vi "_FPGA Check Turbo.vi"(4 "error in":errorcluster) -> (0 "error out":errorcluster, 2 "SpeedOK":bool)   [LabVIEW 2015]
uses:
  Type/_Pump Parameter.ctl
  _RT Global.vi
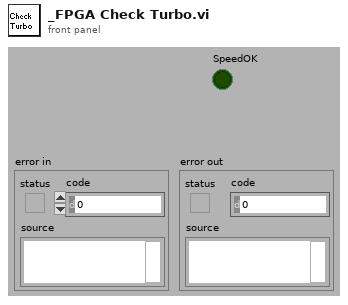
[diagram p1: front panel]
types:
  T1 = typedef "_Pump Parameter.ctl" = enum16{"Turn Pump Motor On", "Turn Pump Motor Off", "Read Pump Oil Deficiency", "Read Rotation Switch Point Attained", "Read Ele. Drive Over Temperature", "Read Pump Over Temperature", "Read Set Rotation Speed Attained", "Read Turbopump Accelerates", "Read Actual Rotation Speed in Hz", "Read Motor Current in A", "Read Operating Hours in h", "Read Motor Voltage in V", "Read Motor Power in W", "Set Rotation Speed Switchpoint in %", "Clear Error", "Read Error Code", "Read Bearing Temperature", "Read Hardware Version", "Read Firmware Version", "Read Operating Hours (Drive)", "Read Rotational Speed (rpm)", "Read Power Stage Temperature", "Read Electronics Temperature", "Read Upper Pump Temperature", "Read Motor Temperature", "Read Error Code History, 1", "Read Error Code History, 2", "Read Error Code History, 3", "Read Error Code History, 4", "Read Error Code History, 5", "Read Error Code History, 6", "Read Error Code History, 7", "Read Error Code History, 8", "Read Error Code History, 9", "Read Error Code History, 10"}
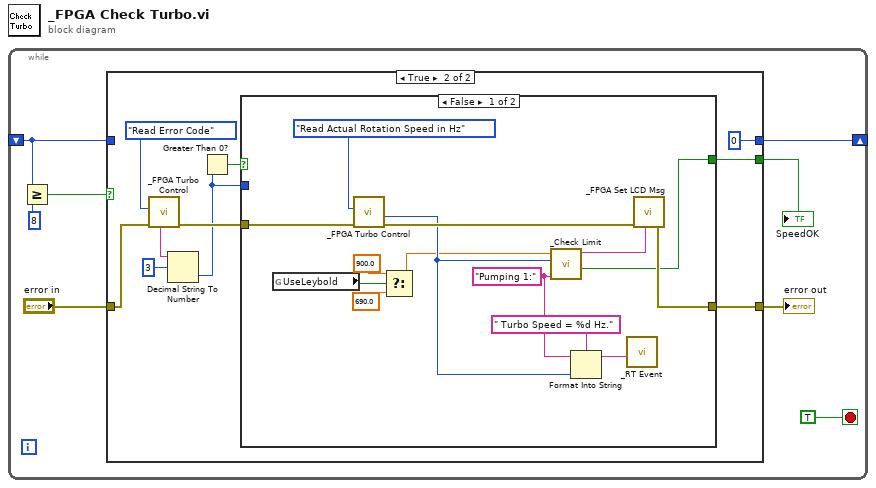
[diagram p0: block diagram]
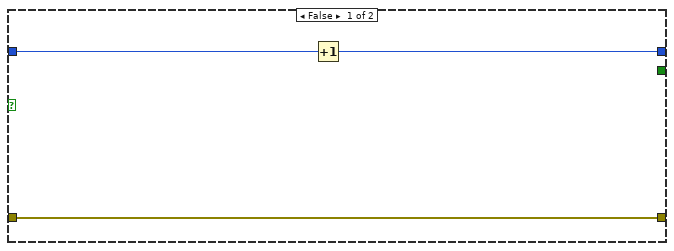
[diagram p2: hidden frame]
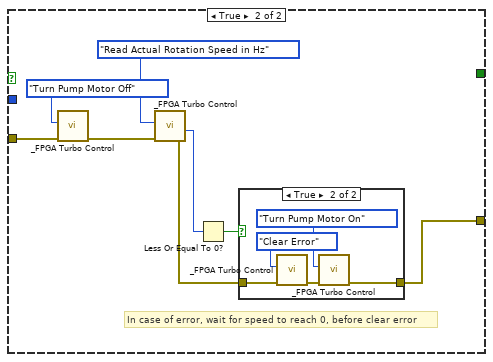
[diagram p3: hidden frame]
diagram:
  n1 = while {
    shift-right: [w7] -> _
    shift-left: _ -> [w5]
    stop <- TRUE stop-if-true
    n2 = Greater Or Equal?(x=w5, y=8) -> (x >= y?=w1:bool)
    n3 = case shown="True" w1 {
      tunnel: [w10 0] -> w7
      tunnel: w5 -> [w11 _]
      tunnel: [w9 w20] -> w3
      tunnel: "error in" -> [w9 w18]
      tunnel: [_ w19] -> w2
      frame False {
        n4 = Increment(x=w11) -> (x+1=w10:i32)
      }
      frame True {
        n5 = call "_FPGA Turbo Control.vi"("error in (no error)"=w18, "Command"=_Pump_Parameter."Read Error Code") -> ("error out"=w17:errorcluster, "Error Code"=w14:string)  [unwired: 2 in, 4 out]
        n6 = Decimal String To Number(string=w14, offset=3 ("offset (0)")) -> (number=w12:i32)  [unwired: 2 out]
        n7 = Greater Than 0?(x=w12) -> (x > 0?=w15:bool)
        n8 = case shown="False" w15 {
          tunnel: [w35 w39] -> w20
          tunnel: [w31 _] -> w19
          tunnel: w17 -> [w30 w38]
          tunnel: w12 -> [_ _]
          frame False {
            w28 = "Pumping 1:" ("Header")
            n9 = global read "_RT Global.vi" "UseLeybold"() -> (w25:bool)
            n10 = call "_FPGA Turbo Control.vi"("error in (no error)"=w30, "Command"=_Pump_Parameter."Read Actual Rotation Speed in Hz") -> ("error out"=w33:errorcluster, "Speed"=w27:i32)  [unwired: 2 in, 4 out]
            n11 = Select(t=900.0 ("Max (100)"), s=w25, f=690.0 ("Max (100)")) -> (s? t:f=w22:dbl)
            n12 = call "_Check Limit.vi"("Header"=w28, "Current"=w27, "Max (100)"=w22) -> ("Max Reached"=w31:bool, "ProgressBar"=w32:string)  [unwired: 1 in, 2 out]
            n13 = Format Into String(format string=" Turbo Speed = %d Hz.", initial string=w28, w27) -> (resulting string=w29:string)  [unwired: 1 in, 1 out]
            n14 = call "_RT Event.vi"("Event"=w29) -> ()  [unwired: 2 in, 5 out]
            n15 = call "_FPGA Set LCD Msg.vi"("Info"=w32, "error in"=w33) -> ("error out"=w35:errorcluster)  [unwired: 5 in, 2 out]
          }
          frame True {
            # "In case of error, wait for speed to reach 0, before clear error"
            n16 = call "_FPGA Turbo Control.vi"("error in (no error)"=w38, "Command"=_Pump_Parameter."Turn Pump Motor Off") -> ("error out"=w37:errorcluster)  [unwired: 2 in, 5 out]
            n17 = call "_FPGA Turbo Control.vi"("error in (no error)"=w37, "Command"=_Pump_Parameter."Read Actual Rotation Speed in Hz") -> ("error out"=w40:errorcluster, "Speed"=w42:i32)  [unwired: 2 in, 4 out]
            n18 = Less Or Equal To 0?(x=w42) -> (x <= 0?=w41:bool)
            n19 = case shown="True" w41 {
              tunnel: w40 -> [w44 w49]
              tunnel: [w44 w45] -> w39
              frame False {
              }
              frame True {
                n20 = call "_FPGA Turbo Control.vi"("error in (no error)"=w49, "Command"=_Pump_Parameter."Clear Error") -> ("error out"=w47:errorcluster)  [unwired: 2 in, 5 out]
                n21 = call "_FPGA Turbo Control.vi"("error in (no error)"=w47, "Command"=_Pump_Parameter."Turn Pump Motor On") -> ("error out"=w45:errorcluster)  [unwired: 2 in, 5 out]
              }
            }
          }
        }
      }
    }
    "error out" <- w3
    "SpeedOK" <- w2
  }
